vi "UHR-Fleezers Control (host) - 12.1.vi"() -> ()   [LabVIEW 2012] (continued)
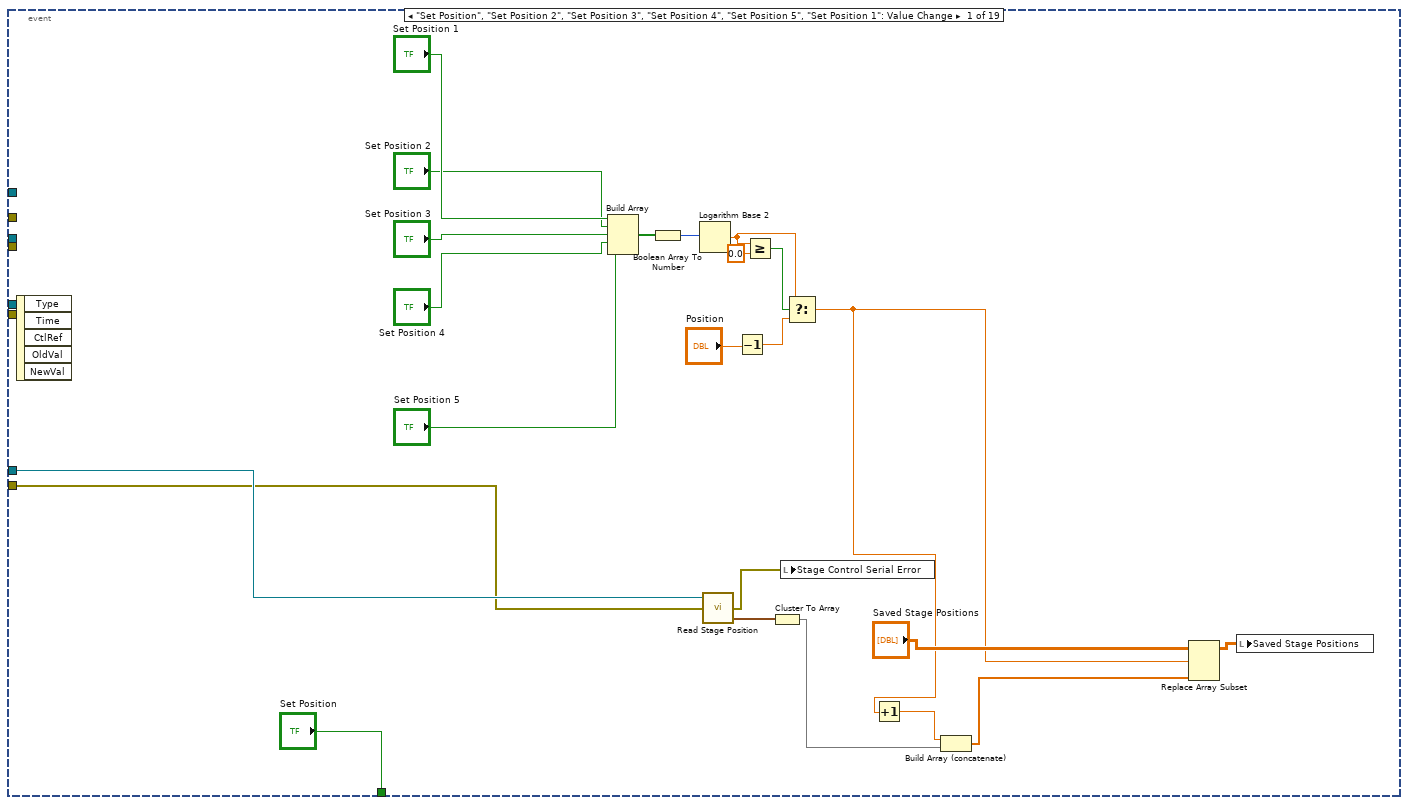
[diagram p3: hidden frame]
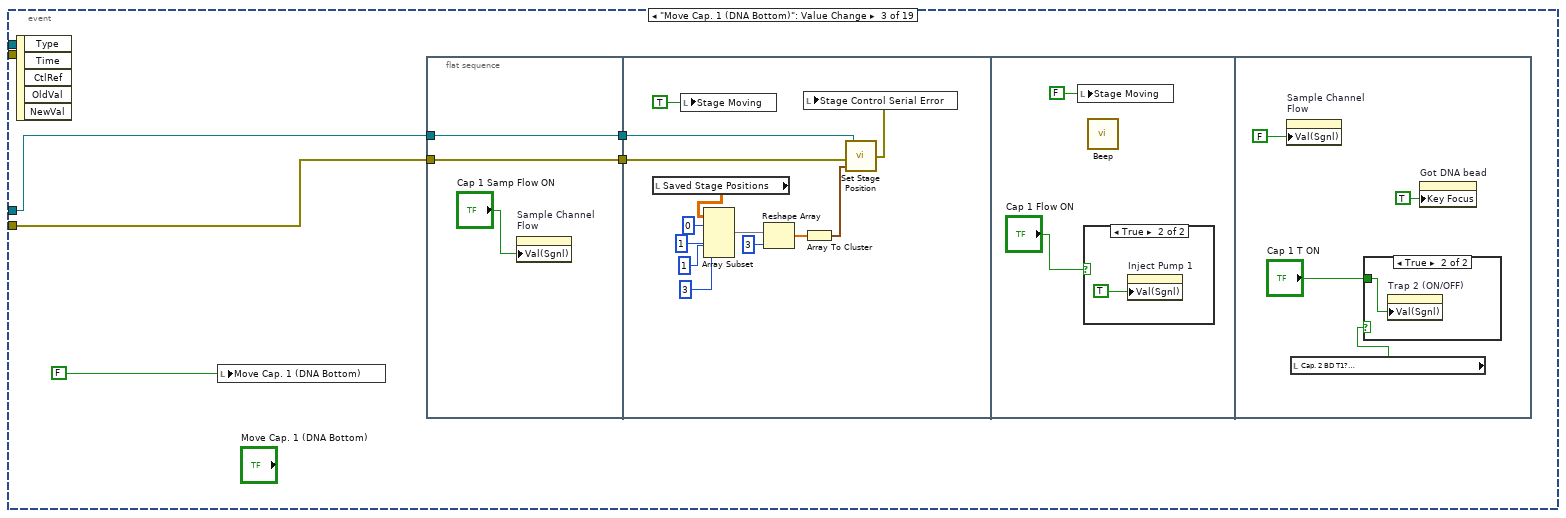
[diagram p4: hidden frame]
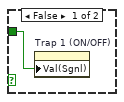
[diagram p6: hidden frame]
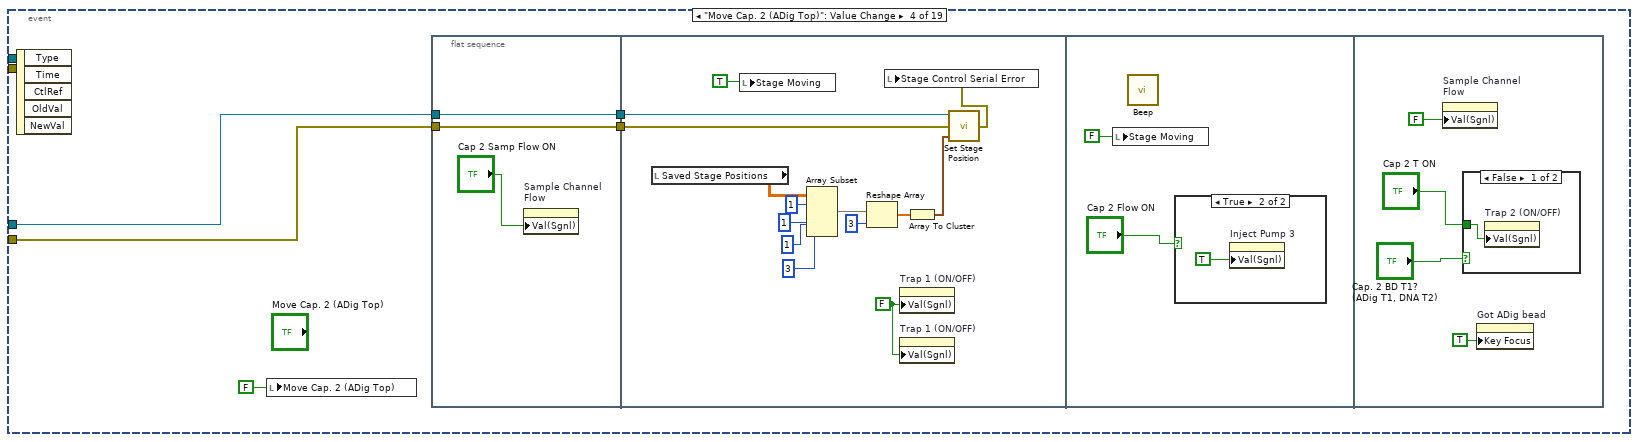
[diagram p7: hidden frame]
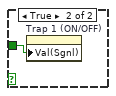
[diagram p9: hidden frame]
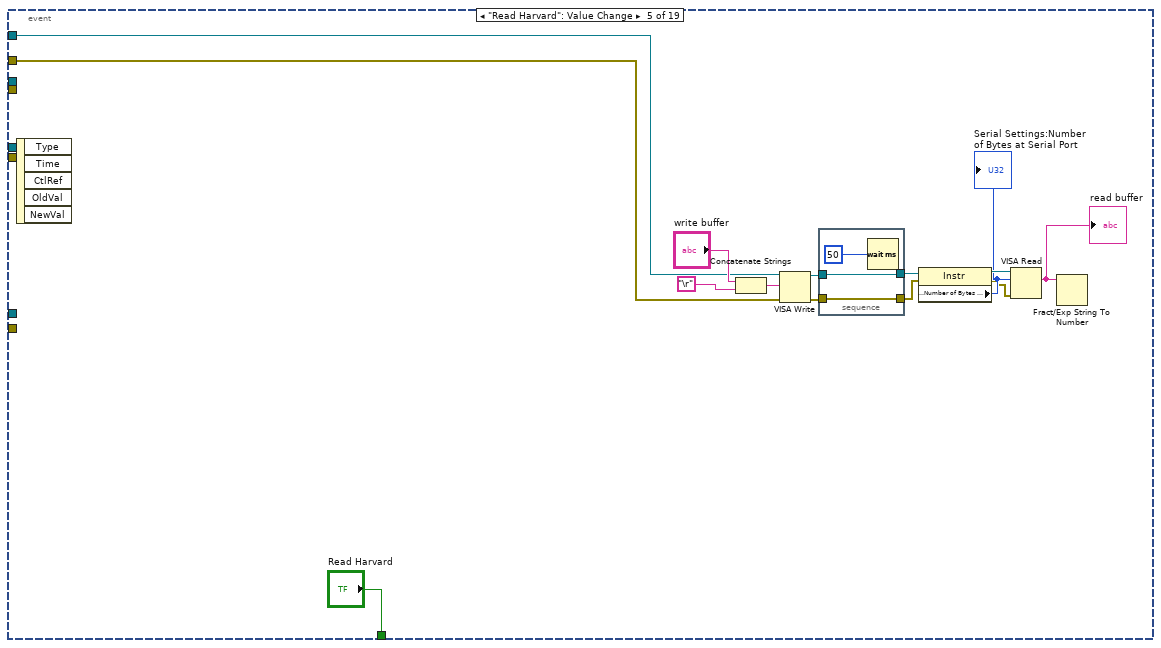
[diagram p10: hidden frame]
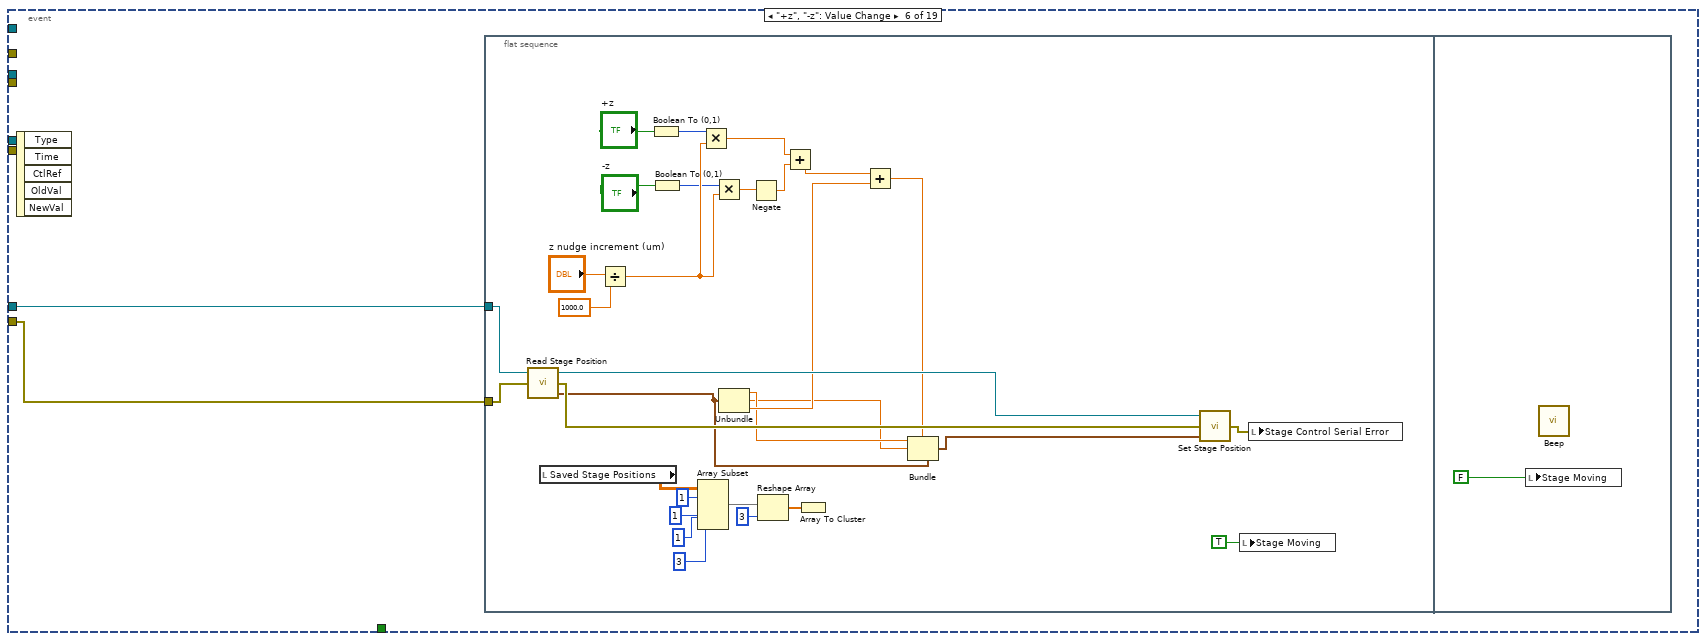
[diagram p11: hidden frame]
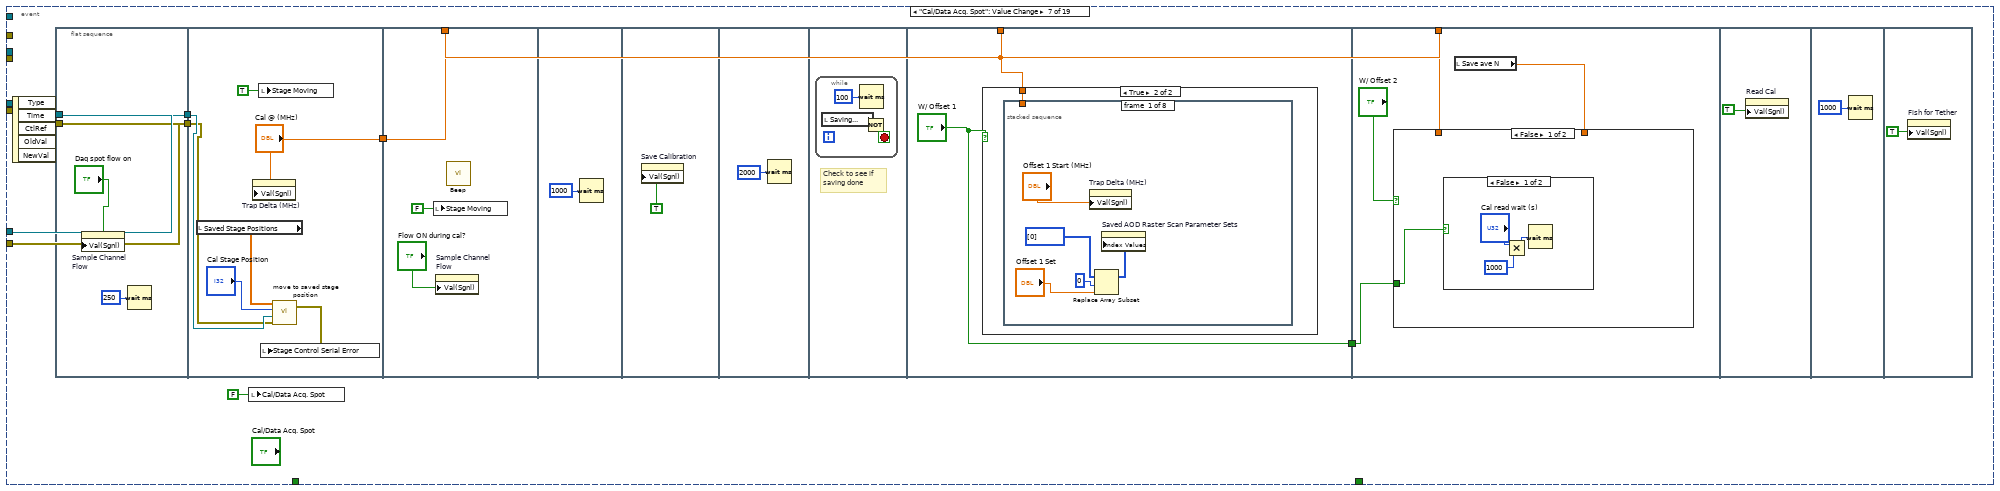
[diagram p12: hidden frame]
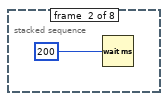
[diagram p14: hidden frame]
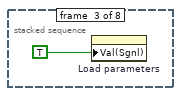
[diagram p15: hidden frame]
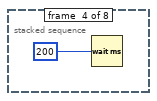
[diagram p16: hidden frame]
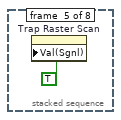
[diagram p17: hidden frame]
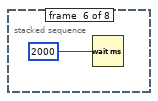
[diagram p18: hidden frame]
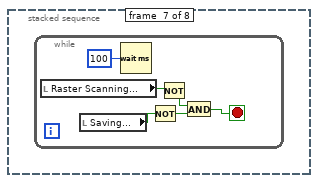
[diagram p19: hidden frame]
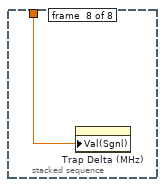
[diagram p20: hidden frame]
                                }
                                frame True {
                                n2885 = local read "Confocal Y 2 (V)"() -> (w4672:dbl)
                                n2886 = local read "Confocal X 2 (V)"() -> (w4671:dbl)
                                n2887 = property on="AO1" class="Slide (strict)"("Val(Sgnl)"=w4672) -> ()  [unwired: 2 in, 2 out]
                                n2888 = property on="AO2" class="Slide (strict)"("Val(Sgnl)"=w4671) -> ()  [unwired: 2 in, 2 out]
                                }
                                }
                                n2889 = case shown="True" w4662 {
                                frame False {
                                }
                                frame True {
                                n2890 = local read "Confocal Y 1 (V)"() -> (w4670:dbl)
                                n2891 = local read "Confocal X 1 (V)"() -> (w4669:dbl)
                                n2892 = property on="AO2" class="Slide (strict)"("Val(Sgnl)"=w4669) -> ()  [unwired: 2 in, 2 out]
                                n2893 = property on="AO1" class="Slide (strict)"("Val(Sgnl)"=w4670) -> ()  [unwired: 2 in, 2 out]
                                }
                                }
                                }
                                }
                                }
                                }
                                }
                                }
                                }
                                }
                                n2894 = local read "Time (s)"() -> (w4607:dbl)
                                n2895 = Subtract(x=w4608, y=w4607) -> (x-y=w4619:dbl)
                                n2896 = Number To Decimal String(number=w4619, width (-)=i16 0) -> (decimal integer string=w4617:string)
                                n2897 = Concatenate Strings(w4617, " s fluorescence event") -> (w4614:string)
                                n2898 = local read "Messages"() -> (w4615:string)
                                n2899 = local write "Duration (s)"(w4619) -> ()
                                n2900 = call "Update messages.vi"("Message to add"=w4614, "Old message string"=w4615) -> ("New message string"=w4613:string)
                                n2901 = local write "Messages"(w4613) -> ()
                                n2902 = call <vilib>:"Beep.vi"() -> ()  [unwired: 12 in]
                                n2903 = local write "Reset Force"(FALSE ("Force Reset")) -> ()
                                n2904 = local write "Fl. High"(TRUE ("Fl. High")) -> ()
                                n2905 = local write "Waiting"(TRUE ("Waiting")) -> ()
                                }
                                }
                                n2906 = node-c288() -> ()  [unwired: 1 in, 1 out]
                                }
                                n2907 = node-c288(w4586) -> ()  [unwired: 1 out]
                                }
                              }
                            }
                          }
                          n2908 = local read "Trap Delta (MHz)"() -> (w4498:dbl)
                          n2909 = local read "Trap Pos FB SP"() -> (w4496:fxp<+/-,16,1>)
                        }
                      }
                    }
                    frame True {
                      n2910 = flat-sequence {
                        tunnel: w4683 -> [w4693]
                        tunnel: [w4693] -> w4687
                        tunnel: w4686 -> [w4692]
                        tunnel: [w4692] -> w4685
                        tunnel: [w4691] -> w4684
                        tunnel: w4682 -> [w4690]
                        tunnel: [w4689] -> w4681
                        tunnel: w4678 -> [w4688]
                        tunnel: [w4688] -> w4677
                        tunnel: w4687 -> [w4763]
                        tunnel: w4685 -> [w4762]
                        tunnel: w4684 -> [w4761]
                        tunnel: w4681 -> [w4760]
                        tunnel: w4677 -> [w4759]
                        tunnel: [w4760] -> w4680
                        frame #0 {
                          n2911 = call <vilib>:"Beep.vi"() -> ()  [unwired: 3 in, 9 out]
                          n2912 = local write "Waiting"(FALSE ("Waiting")) -> ()
                          n2913 = Increment(x=w4690) -> (x+1=w4689:u8)
                          n2914 = case shown="\"Yank\"" w4692 {
                            tunnel: w4689 -> [_ _ w4699]
                            frame "Image" {
                              n2915 = property on="Confocal Image" class="Bool (strict)"("Val(Sgnl)"=TRUE ("Value (Signaling)")) -> ()  [unwired: 2 in, 2 out]
                            }
                            frame "Alarm", Default {
                            }
                            frame "Yank" {
                              n2916 = flat-sequence {
                                tunnel: w4699 -> [w4702]
                                tunnel: [w4701] -> w4698
                                tunnel: ["N Array El"] -> w4697
                                tunnel: w4698 -> [w4716]
                                tunnel: w4697 -> [w4712]
                                frame #0 {
                                n2917 = Multiply(x="Yank Delay (s)", y=1000.0) -> (x*y=w4705:dbl)
                                n2918 = Quotient & Remainder(x=w4702, y="N Array El") -> (x-y*floor(x/y)=w4701:u8)  [unwired: 1 out]
                                n2919 = Wait (ms)(milliseconds to wait=w4705) -> ()  [unwired: 1 out]
                                }
                                frame #1 {
                                n2920 = Random Number (0-1)() -> (number: 0 to 1=w4713:dbl)
                                n2921 = Multiply(x=w4712, y=w4713) -> (x*y=w4711:dbl)
                                n2922 = Round Toward -Infinity(1:w4711) -> (0:w4710:dbl)
                                n2923 = Select(t=w4710, s="Random Choice", f=w4716) -> (s? t:f=w4714:dbl)
                                n2924 = Select(t="Yank to Trap Delta (MHz)", s="Yank to which?", f="Yank to SP") -> (s? t:f=w4707:dbl[])
                                n2925 = Index Array(array=w4707, index=w4714) -> (element=w4717:dbl)
                                n2926 = case shown="False" "Yank to which?" {
                                tunnel: w4717 -> [w4718 w4744]
                                frame False {
                                n2927 = flat-sequence {
                                tunnel: w4718 -> [w4719]
                                frame #0 {
                                n2928 = property on="Trap Pos FB SP" class="DigNum (strict)"("Val(Sgnl)"=w4719) -> ()  [unwired: 2 in, 2 out]
                                }
                                frame #1 {
                                n2929 = Wait (ms)(milliseconds to wait=u32 700) -> ()  [unwired: 1 out]
                                }
                                frame #2 {
                                n2930 = local read "Action (%)"() -> (w4724:dbl)
                                n2931 = Absolute Value(x=w4724) -> (abs(x)=w4723:dbl)
                                n2932 = Greater?(x=w4723, y=70.0) -> (0:w4721:bool)
                                n2933 = property on="Remove Action Offset" class="Bool (strict)"("Val(Sgnl)"=w4721) -> ()  [unwired: 2 in, 2 out]
                                }
                                frame #3 {
                                n2934 = for {
                                N: 4 -> [_]
                                n2935 = flat-sequence {
                                frame #0 {
                                n2936 = Wait (ms)(milliseconds to wait=u32 500) -> ()  [unwired: 1 out]
                                }
                                frame #1 {
                                n2937 = local read "Action (%)"() -> (w4730:dbl)
                                n2938 = Absolute Value(x=w4730) -> (abs(x)=w4729:dbl)
                                n2939 = Greater?(x=w4729, y=70.0) -> (0:w4727:bool)
                                n2940 = property on="Remove Action Offset" class="Bool (strict)"("Val(Sgnl)"=w4727) -> ()  [unwired: 2 in, 2 out]
                                }
                                }
                                }
                                }
                                frame #4 {
                                n2941 = local read "Shift confocal"() -> (w4734:bool)
                                n2942 = local read "Mean"() -> (w4737:dbl)
                                n2943 = Greater?(x=w4737, y=11.0) -> (0:w4733:bool)
                                n2944 = Not(x=w4733) -> (.not. x?=w4732:bool)
                                n2945 = And(x=w4732, y=w4734) -> (x .and. y?=w4731:bool)
                                n2946 = And(x=w4733, y=w4734) -> (x .and. y?=w4735:bool)
                                n2947 = case shown="True" w4735 {
                                frame False {
                                }
                                frame True {
                                n2948 = local read "Confocal X 2 (V)"() -> (w4740:dbl)
                                n2949 = local read "Confocal Y 2 (V)"() -> (w4741:dbl)
                                n2950 = property on="AO2" class="Slide (strict)"("Val(Sgnl)"=w4740) -> ()  [unwired: 2 in, 2 out]
                                n2951 = property on="AO1" class="Slide (strict)"("Val(Sgnl)"=w4741) -> ()  [unwired: 2 in, 2 out]
                                }
                                }
                                n2952 = case shown="True" w4731 {
                                frame False {
                                }
                                frame True {
                                n2953 = local read "Confocal X 1 (V)"() -> (w4738:dbl)
                                n2954 = local read "Confocal Y 1 (V)"() -> (w4739:dbl)
                                n2955 = property on="AO1" class="Slide (strict)"("Val(Sgnl)"=w4739) -> ()  [unwired: 2 in, 2 out]
                                n2956 = property on="AO2" class="Slide (strict)"("Val(Sgnl)"=w4738) -> ()  [unwired: 2 in, 2 out]
                                }
                                }
                                }
                                frame #5 {
                                n2957 = Wait (ms)(milliseconds to wait=u32 1500) -> ()  [unwired: 1 out]
                                }
                                frame #6 {
                                n2958 = property on="Rem fb disp offset" class="Bool (strict)"("Val(Sgnl)"=TRUE ("Value (Signaling)")) -> ()  [unwired: 2 in, 2 out]
                                }
                                }
                                }
                                frame True {
                                n2959 = flat-sequence {
                                tunnel: w4744 -> [w4745]
                                frame #0 {
                                n2960 = property on="Trap Delta (MHz)" class="DigNum (strict)"("Val(Sgnl)"=w4745) -> ()  [unwired: 2 in, 2 out]
                                }
                                frame #1 {
                                n2961 = Wait (ms)(milliseconds to wait=u32 500) -> ()  [unwired: 1 out]
                                }
                                frame #2 {
                                n2962 = local read "Shift confocal"() -> (w4749:bool)
                                n2963 = local read "Mean"() -> (w4747:dbl)
                                n2964 = Greater?(x=w4747, y=11.0) -> (0:w4750:bool)
                                n2965 = Not(x=w4750) -> (.not. x?=w4751:bool)
                                n2966 = And(x=w4751, y=w4749) -> (x .and. y?=w4753:bool)
                                n2967 = And(x=w4750, y=w4749) -> (x .and. y?=w4752:bool)
                                n2968 = case shown="True" w4752 {
                                frame False {
                                }
                                frame True {
                                n2969 = local read "Confocal Y 2 (V)"() -> (w4757:dbl)
                                n2970 = local read "Confocal X 2 (V)"() -> (w4756:dbl)
                                n2971 = property on="AO1" class="Slide (strict)"("Val(Sgnl)"=w4757) -> ()  [unwired: 2 in, 2 out]
                                n2972 = property on="AO2" class="Slide (strict)"("Val(Sgnl)"=w4756) -> ()  [unwired: 2 in, 2 out]
                                }
                                }
                                n2973 = case shown="True" w4753 {
                                frame False {
                                }
                                frame True {
                                n2974 = local read "Confocal X 1 (V)"() -> (w4754:dbl)
                                n2975 = local read "Confocal Y 1 (V)"() -> (w4755:dbl)
                                n2976 = property on="AO2" class="Slide (strict)"("Val(Sgnl)"=w4754) -> ()  [unwired: 2 in, 2 out]
                                n2977 = property on="AO1" class="Slide (strict)"("Val(Sgnl)"=w4755) -> ()  [unwired: 2 in, 2 out]
                                }
                                }
                                }
                                }
                                }
                                }
                                }
                              }
                            }
                          }
                          n2978 = local read "Time (s)"() -> (w4691:dbl)
                          "Fl. High" <- TRUE ("Yanking")
                        }
                        frame #1 {
                          n2979 = local read "Auto F Reset"() -> (w4758:bool)
                          n2980 = case shown="True" w4758 {
                            tunnel: w4763 -> [_ w4767]
                            tunnel: w4762 -> [_ w4766]
                            tunnel: w4761 -> [_ w4765]
                            tunnel: w4759 -> [_ w4764]
                            frame False {
                            }
                            frame True {
                              n2981 = node-c288() -> (w4769:T20)  [unwired: 4 out]
                              n2982 = timed-loop {
                                timing: w4769 -> [_]
                                timing-out: [_] -> w4768
                                tunnel: w4767 -> [w4787]
                                tunnel: w4766 -> [w4786]
                                tunnel: w4765 -> [w4785]
                                tunnel: w4764 -> [w4784]
                                stop <- w4770 stop-if-true
                                n2983 = node-c288() -> ()  [unwired: 2 out]
                                n2984 = local read "Fl. Delta Thresh. (kHz)"() -> (w4778:dbl)
                                n2985 = local read "Fl. Triggered..."() -> (w4783:bool)
                                n2986 = local read "Delta Fl. 1"() -> (w4774:dbl)
                                n2987 = local read "Delta Fl. 2"() -> (w4772:dbl)
                                n2988 = local read "Stop All"() -> (w4781:bool)
                                n2989 = local read "APD to Watch"() -> (w4773:bool)
                                n2990 = Select(t=w4774, s=w4773, f=w4772) -> (s? t:f=w4771:dbl)
                                n2991 = Not(x=w4783) -> (.not. x?=w4782:bool)
                                n2992 = Multiply(x=w4778, y=1000.0) -> (x*y=w4777:dbl)
                                n2993 = Negate(x=w4777) -> (-x=w4776:dbl)
                                n2994 = Less?(x=w4771, y=w4776) -> (x < y?=w4780:bool)
                                n2995 = Compound Arithmetic op=OR(w4780, w4781, w4782, "Reset Force") -> (w4770:bool)
                                n2996 = case shown="True" w4770 {
                                tunnel: w4787 -> [_ w4802]
                                tunnel: w4786 -> [_ w4801]
                                tunnel: w4785 -> [_ w4791]
                                tunnel: w4784 -> [_ w4793]
                                frame False {
                                }
                                frame True {
                                n2997 = local read "Time (s)"() -> (w4792:dbl)
                                n2998 = case shown="\"Yank\"" w4801 {
                                tunnel: w4802 -> [_ w4805]
                                tunnel: w4793 -> [_ w4803]
                                frame "Image", Default {
                                }
                                frame "Yank" {
                                n2999 = flat-sequence {
                                tunnel: [w4811] -> w4806
                                tunnel: w4805 -> [w4811]
                                tunnel: [w4807] -> w4804
                                tunnel: w4803 -> [w4807]
                                tunnel: w4806 -> [w4814]
                                tunnel: w4804 -> [w4812]
                                frame #0 {
                                n3000 = local read "Yank Delay (s)"() -> (w4810:dbl)
                                n3001 = Multiply(x=w4810, y=1000.0) -> (x*y=w4808:dbl)
                                n3002 = Wait (ms)(milliseconds to wait=w4808) -> ()  [unwired: 1 out]
                                }
                                frame #1 {
                                n3003 = local read "Yank to which?"() -> (w4813:bool)
                                n3004 = case shown="False" w4813 {
                                tunnel: w4814 -> [_ w4841]
                                tunnel: w4812 -> [w4815 _]
                                frame False {
                                n3005 = flat-sequence {
                                tunnel: w4815 -> [w4816]
                                frame #0 {
                                n3006 = property on="Trap Pos FB SP" class="DigNum (strict)"("Val(Sgnl)"=w4816) -> ()  [unwired: 2 in, 2 out]
                                }
                                frame #1 {
                                n3007 = Wait (ms)(milliseconds to wait=u32 700) -> ()  [unwired: 1 out]
                                }
                                frame #2 {
                                n3008 = local read "Action (%)"() -> (w4821:dbl)
                                n3009 = Absolute Value(x=w4821) -> (abs(x)=w4820:dbl)
                                n3010 = Greater?(x=w4820, y=70.0) -> (0:w4818:bool)
                                n3011 = property on="Remove Action Offset" class="Bool (strict)"("Val(Sgnl)"=w4818) -> ()  [unwired: 2 in, 2 out]
                                }
                                frame #3 {
                                n3012 = for {
                                N: 4 -> [_]
                                n3013 = flat-sequence {
                                frame #0 {
                                n3014 = Wait (ms)(milliseconds to wait=u32 500) -> ()  [unwired: 1 out]
                                }
                                frame #1 {
                                n3015 = local read "Action (%)"() -> (w4827:dbl)
                                n3016 = Absolute Value(x=w4827) -> (abs(x)=w4826:dbl)
                                n3017 = Greater?(x=w4826, y=70.0) -> (0:w4824:bool)
                                n3018 = property on="Remove Action Offset" class="Bool (strict)"("Val(Sgnl)"=w4824) -> ()  [unwired: 2 in, 2 out]
                                }
                                }
                                }
                                }
                                frame #4 {
                                n3019 = local read "Shift confocal"() -> (w4832:bool)
                                n3020 = local read "Mean"() -> (w4834:dbl)
                                n3021 = Greater?(x=w4834, y=11.0) -> (0:w4831:bool)
                                n3022 = Not(x=w4831) -> (.not. x?=w4830:bool)
                                n3023 = And(x=w4831, y=w4832) -> (x .and. y?=w4829:bool)
                                n3024 = And(x=w4830, y=w4832) -> (x .and. y?=w4828:bool)
                                n3025 = case shown="True" w4829 {
                                frame False {
                                }
                                frame True {
                                n3026 = local read "Confocal Y 2 (V)"() -> (w4838:dbl)
                                n3027 = local read "Confocal X 2 (V)"() -> (w4837:dbl)
                                n3028 = property on="AO2" class="Slide (strict)"("Val(Sgnl)"=w4837) -> ()  [unwired: 2 in, 2 out]
                                n3029 = property on="AO1" class="Slide (strict)"("Val(Sgnl)"=w4838) -> ()  [unwired: 2 in, 2 out]
                                }
                                }
                                n3030 = case shown="True" w4828 {
                                frame False {
                                }
                                frame True {
                                n3031 = local read "Confocal X 1 (V)"() -> (w4835:dbl)
                                n3032 = local read "Confocal Y 1 (V)"() -> (w4836:dbl)
                                n3033 = property on="AO1" class="Slide (strict)"("Val(Sgnl)"=w4836) -> ()  [unwired: 2 in, 2 out]
                                n3034 = property on="AO2" class="Slide (strict)"("Val(Sgnl)"=w4835) -> ()  [unwired: 2 in, 2 out]
                                }
                                }
                                }
                                frame #5 {
                                n3035 = Wait (ms)(milliseconds to wait=u32 1500) -> ()  [unwired: 1 out]
                                }
                                frame #6 {
                                n3036 = property on="Rem fb disp offset" class="Bool (strict)"("Val(Sgnl)"=TRUE ("Value (Signaling)")) -> ()  [unwired: 2 in, 2 out]
                                }
                                }
                                }
                                frame True {
                                n3037 = flat-sequence {
                                tunnel: w4841 -> [w4842]
                                frame #0 {
                                n3038 = property on="Trap Delta (MHz)" class="DigNum (strict)"("Val(Sgnl)"=w4842) -> ()  [unwired: 2 in, 2 out]
                                }
                                frame #1 {
                                n3039 = Wait (ms)(milliseconds to wait=u32 500) -> ()  [unwired: 1 out]
                                }
                                frame #2 {
                                n3040 = local read "Shift confocal"() -> (w4848:bool)
                                n3041 = local read "Mean"() -> (w4850:dbl)
                                n3042 = Greater?(x=w4850, y=11.0) -> (0:w4847:bool)
                                n3043 = Not(x=w4847) -> (.not. x?=w4846:bool)
                                n3044 = And(x=w4847, y=w4848) -> (x .and. y?=w4845:bool)
                                n3045 = And(x=w4846, y=w4848) -> (x .and. y?=w4844:bool)
                                n3046 = case shown="True" w4845 {
                                frame False {
                                }
                                frame True {
                                n3047 = local read "Confocal Y 2 (V)"() -> (w4854:dbl)
                                n3048 = local read "Confocal X 2 (V)"() -> (w4853:dbl)
                                n3049 = property on="AO2" class="Slide (strict)"("Val(Sgnl)"=w4853) -> ()  [unwired: 2 in, 2 out]
                                n3050 = property on="AO1" class="Slide (strict)"("Val(Sgnl)"=w4854) -> ()  [unwired: 2 in, 2 out]
                                }
                                }
                                n3051 = case shown="True" w4844 {
                                frame False {
                                }
                                frame True {
                                n3052 = local read "Confocal Y 1 (V)"() -> (w4852:dbl)
                                n3053 = local read "Confocal X 1 (V)"() -> (w4851:dbl)
                                n3054 = property on="AO2" class="Slide (strict)"("Val(Sgnl)"=w4851) -> ()  [unwired: 2 in, 2 out]
                                n3055 = property on="AO1" class="Slide (strict)"("Val(Sgnl)"=w4852) -> ()  [unwired: 2 in, 2 out]
                                }
                                }
                                }
                                }
                                }
                                }
                                }
                                }
                                }
                                }
                                n3056 = local read "Messages"() -> (w4800:string)
                                n3057 = Subtract(x=w4792, y=w4791) -> (x-y=w4798:dbl)
                                "Duration (s)" <- w4798
                                n3058 = Number To Decimal String(number=w4798, width (-)=i16 0) -> (decimal integer string=w4796:string)
                                n3059 = Concatenate Strings(w4796, " s fluorescence event." ("string")) -> (w4794:string)
                                n3060 = call "Update messages.vi"("Message to add"=w4794, "Old message string"=w4800) -> ("New message string"=w4799:string)
                                n3061 = local write "Reset Force"(FALSE ("Reset Force")) -> ()
                                n3062 = local write "Waiting"(TRUE ("Waiting")) -> ()
                                n3063 = local write "Messages"(w4799) -> ()
                                n3064 = local write "Fl. High"(FALSE ("Fl. High")) -> ()
                                n3065 = call <vilib>:"Beep.vi"() -> ()  [unwired: 3 in, 9 out]
                                }
                                }
                                n3066 = node-c288() -> ()  [unwired: 2 out]
                              }
                              n3067 = node-c288(w4768) -> ()  [unwired: 1 out]
                            }
                          }
                        }
                      }
                      n3068 = local read "Trap Delta (MHz)"() -> (w4683:dbl)
                      n3069 = local read "Trap Pos FB SP"() -> (w4678:fxp<+/-,16,1>)
                    }
                  }
                }
                frame #1 {
                  n3070 = local read "Stop All"() -> (w4864:bool)
                  n3071 = local read "Fl. Triggered..."() -> (w4862:bool)
                  n3072 = Not(x=w4862) -> (.not. x?=w4863:bool)
                  n3073 = Or(x=w4863, y=w4864) -> (x .or. y?=w4861:bool)
                }
              }
              n3074 = case shown="True" w4455 {
                frame False {
                }
                frame True {
                  n3075 = local read "Confocal Y 1 (V)"() -> (w4465:dbl)
                  n3076 = local read "Confocal X 1 (V)"() -> (w4464:dbl)
                  n3077 = property on="AO2" class="Slide (strict)"("Val(Sgnl)"=w4464) -> ()  [unwired: 2 in, 2 out]
                  n3078 = property on="AO1" class="Slide (strict)"("Val(Sgnl)"=w4465) -> ()  [unwired: 2 in, 2 out]
                }
              }
              n3079 = case shown="True" w4455 {
                frame False {
                }
                frame True {
                  w4463 = FALSE ("Fl. High")
                  n3080 = local write "Waiting"(w4463) -> ()
                  n3081 = local write "Fl. High"(w4463) -> ()
                }
              }
              n3082 = node-c288() -> ()  [unwired: 2 out]
            }
            n3083 = node-c288(w4453) -> ()  [unwired: 1 out]
          }
        }
      }
      event "Stop All": Value Change {
        n3084 = event-data() -> ()  [unwired: 7 out]
        n3085 = local read "Stop All"() -> (w4869:bool)
      }
    }
    n3086 = node-c288() -> ()  [unwired: 2 out]
  }
  n3087 = node-c288(w115) -> ()  [unwired: 1 out]
  n3088 = node-c288(w117) -> ()  [unwired: 1 out]
  n3089 = node-c288(w102) -> ()  [unwired: 1 out]
  n3090 = property on="Saved trap pos" class="WFGraph (strict)"("Visible"=FALSE) -> ()  [unwired: 2 in, 2 out]
  n3091 = property on="Trap Delta Graph" class="WFGraph (strict)"("Visible"=TRUE) -> ()  [unwired: 2 in, 2 out]
  n3092 = local write "Trap pos"(FALSE ("Trap pos")) -> ()
  n3093 = local write "Offset (nm)"(0.0 ("Offset (nm)")) -> ()
  n3094 = local write "Bead Mean (nm)"(0.0 ("Bead Mean (nm)")) -> ()
  n3095 = disable-structure shown="Disabled" {
    disable-tunnel: w106 -> [w4871 _]
    disable-tunnel: w105 -> [w4870 _]
    frame Disabled {
      n3096 = VISA Close(VISA resource name=w4871, error in (no error)=w4870) -> (error out=w4872:errorcluster)
      n3097 = call <vilib>:"Simple Error Handler.vi"("error in (no error)"=w4872) -> ()  [unwired: 1 in, 8 out]
    }
    frame Enabled {
    }
  }
  n3098 = node-c288(w193) -> ()  [unwired: 1 out]
  n3099 = node-c288(w113) -> ()  [unwired: 1 out]
  n3100 = flat-sequence {
    tunnel: w284 -> [w4876]
    tunnel: w286 -> [w4877]
    tunnel: [w4875] -> w265
    tunnel: [w4874] -> w264
    tunnel: w249 -> [_]
    tunnel: w201 -> [_]
    tunnel: w119 -> [_]
    tunnel: w265 -> [w4878]
    tunnel: w264 -> [w4879]
    frame #0 {
      w4873 = FALSE ("AI to FIFO")
      n3101 = xnode "Read/Write Control"("FPGA VI Reference In"=w4877, "error in"=w4876, "AI to FIFO"=w4873, "APD to FIFO"=w4873) -> ("FPGA VI Reference Out"=w4875:T18, "error out"=w4874:errorcluster)
    }
    frame #1 {
      n3102 = xnode "Close FPGA VI Reference"("FPGA VI Reference In"=w4878, "error in"=w4879) -> ("error out"=→"error out":errorcluster)
    }
  }
